vi "FP_Get Control Properties.vi"(8 "Error":errorcluster, 11 "Ctrl":refnum<vi>) -> (0 "Error Out":errorcluster, 1 "ClassName Out":string, 2 "Label.Text Out":string, 3 "Ctl Refnum Out":refnum<vi>)   [LabVIEW 2020]
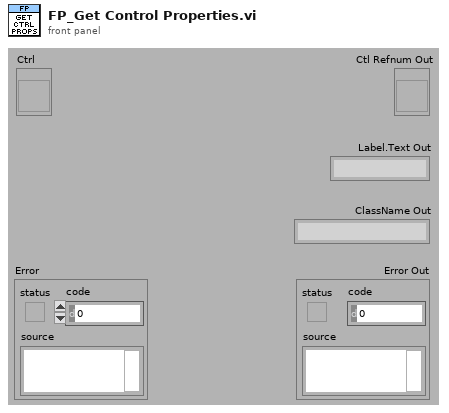
[diagram p1: front panel]
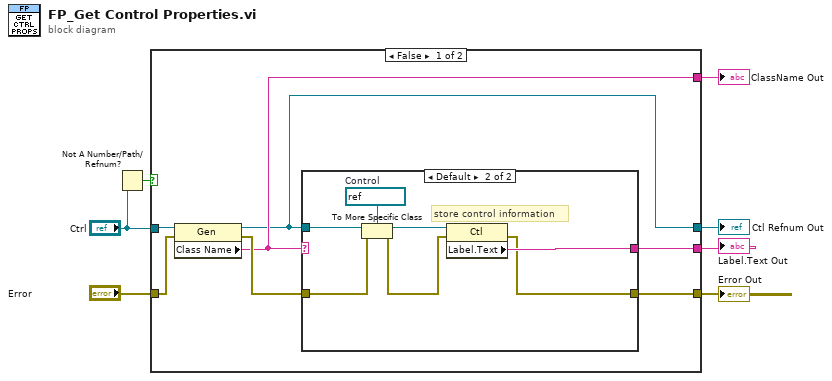
[diagram p0: block diagram]
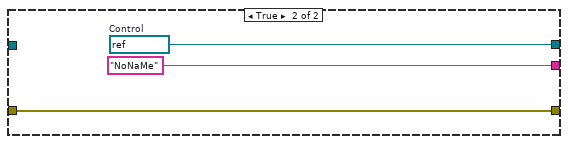
[diagram p3: hidden frame]
diagram:
  n1 = Not A Number/Path/Refnum?(number/path/refnum="Ctrl") -> (NaN/Path/Refnum?=w2:bool)
  n2 = case shown="False" w2 {
    tunnel: "Ctrl" -> [w14 _]
    tunnel: [w8 w23] -> w7
    tunnel: [w13 "NoNaMe" ("t")] -> w6
    tunnel: [w12 w24] -> w5
    tunnel: "Error" -> [w10 w24]
    tunnel: [w9 _] -> w1
    frame False {
      n3 = property class="Gen"(reference=w14, error in=w10) -> (reference out=w8:refnum<vi>, error out=w11:errorcluster, "Class Name"=w9:string)
      n4 = case shown="Default" w9 {
        tunnel: [_ w22] -> w13
        tunnel: [w15 w21] -> w12
        tunnel: w11 -> [w15 w18]
        tunnel: w8 -> [_ w20]
        frame "Page" {
        }
        frame Default {
          w16 = refnum<vi> refnum  # Control
          # "store control information"
          n5 = To More Specific Class(target class=w16, reference=w20, error in=w18) -> (specific class reference=w19:refnum<vi>, error out=w17:errorcluster)
          n6 = property class="Ctl"(reference=w19, error in=w17) -> (error out=w21:errorcluster, "Label.Text"=w22:string)  [unwired: 1 out]
        }
      }
    }
    frame True {
      w23 = refnum<vi> refnum  # Control
    }
  }
  "Ctl Refnum Out" <- w7
  "Label.Text Out" <- w6
  "Error Out" <- w5
  "ClassName Out" <- w1
